vi "Liste-maker.vi"(1 "Path":path) -> (0 "Save Path":path)   [LabVIEW 2019]
panel:
  in  "load":bool
  in  "cancel":bool
  in  "Apperçu_ghost":string[][](table)=[["1", "NGC1", "1:00:00", "0:00:00", "2000"], ["2", "NGC2", "2:00:00", "-1:00:00", "2000"], ["3", "NGC3", "3:00:00", "-2:00:00", "2000"], ["4", "NGC4", "4:00:00", "-3:00:00", "2000"], ["5", "NGC5", "5:00:00", "-4:00:00", "2000"]]
  in  "i":string
  in  "reorder":bool
  in  "erase":bool
  in  "add":bool
  in  "Epoch":string
  in  "DEC":string
  in  "RA":string
  in  "Pseudonyme":string
  out "tmp_str":string
  in  "save":bool
  in  "stop":bool
  out "Apperçu":string[][](table)=[["1", "NGC1", "1:00:00", "0:00:00", "2000"], ["2", "NGC2", "2:00:00", "-1:00:00", "2000"], ["3", "NGC3", "3:00:00", "-2:00:00", "2000"], ["4", "NGC4", "4:00:00", "-3:00:00", "2000"], ["5", "NGC5", "5:00:00", "-4:00:00", "2000"]]
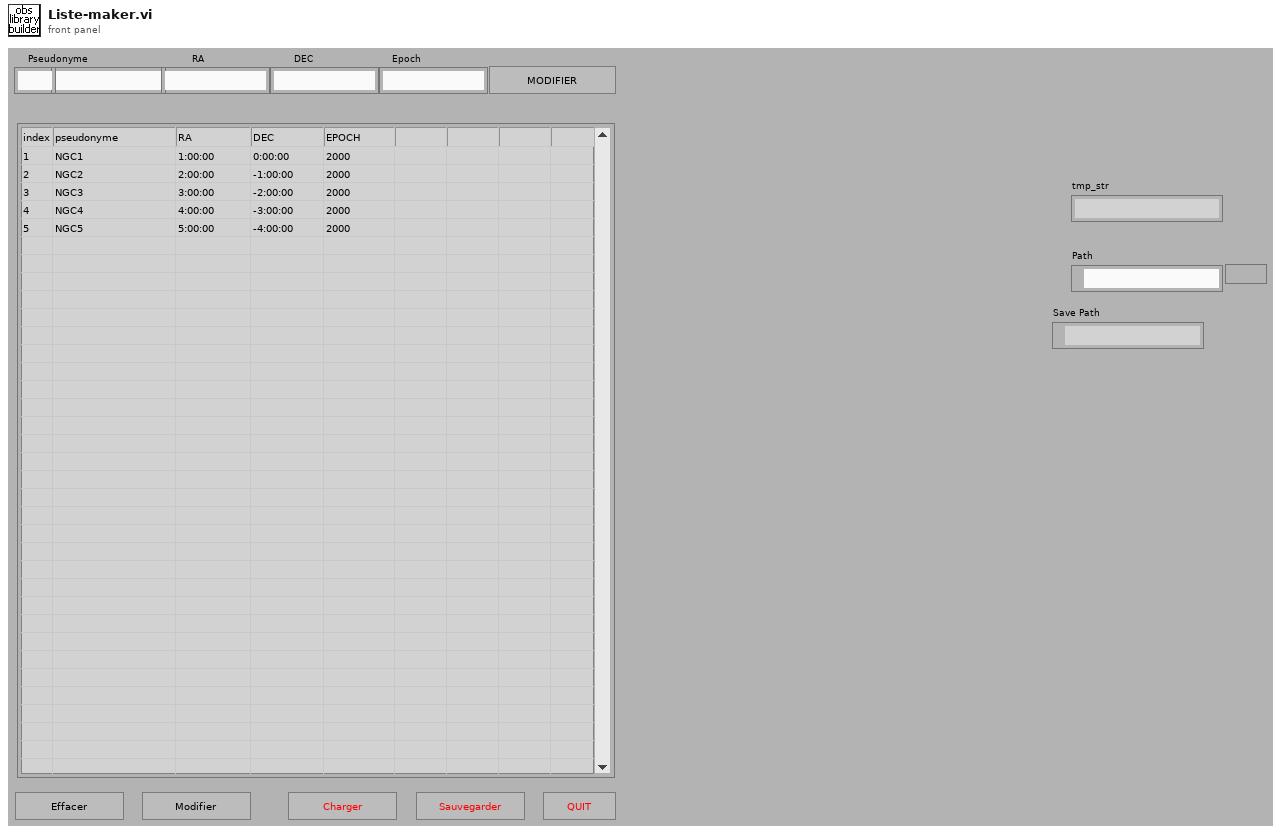
[diagram p1: front panel]
types:
  T1 = typedef "LVRowAndColumnTypeDef.ctl" = cluster{"Row":i32, "Column":i32}
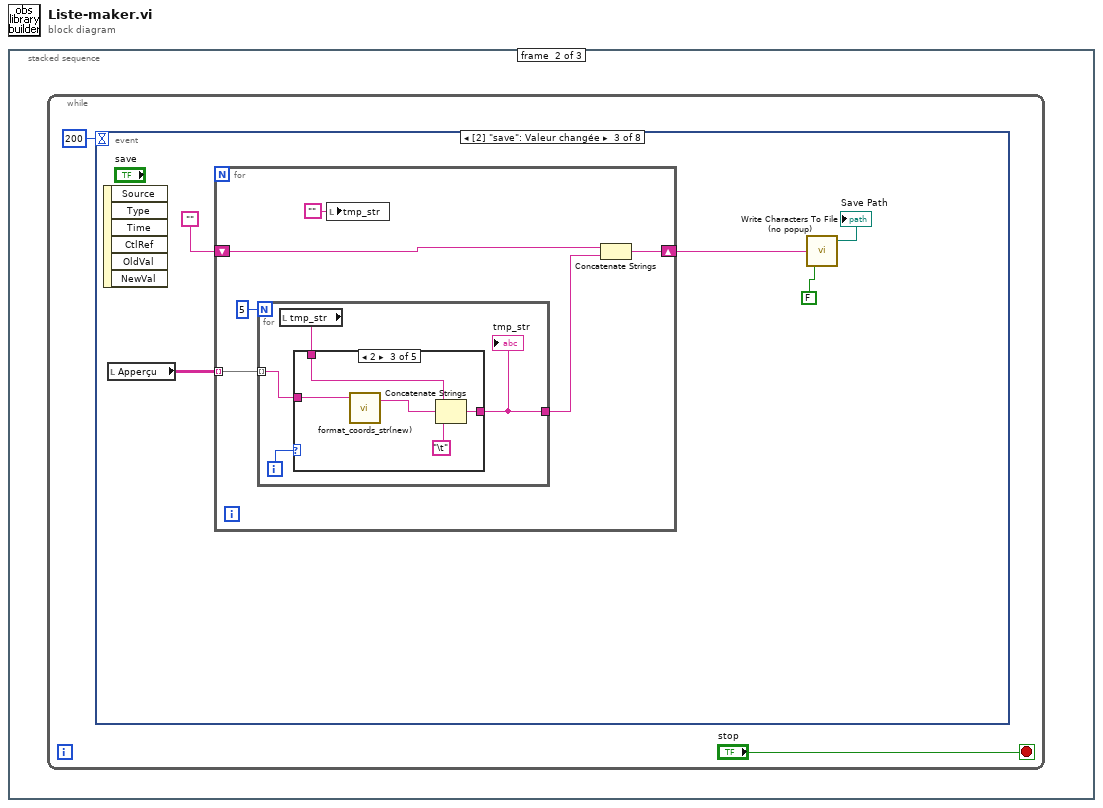
[diagram p0: block diagram]
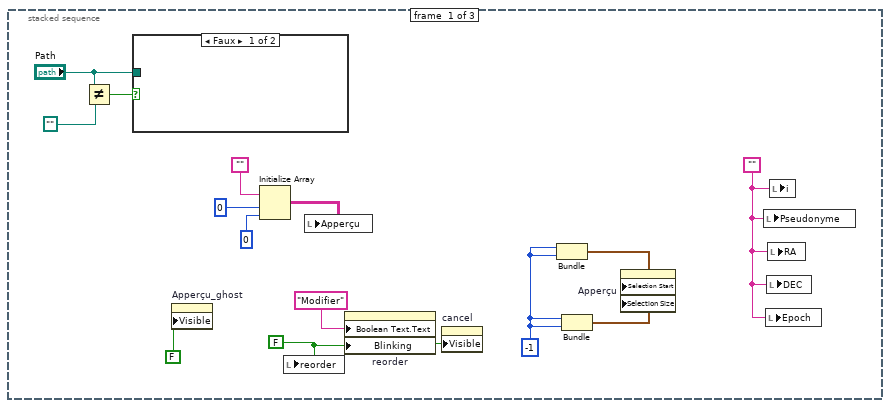
[diagram p2: hidden frame]
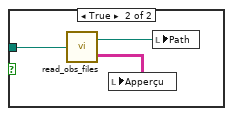
[diagram p3: hidden frame]
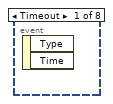
[diagram p4: hidden frame]
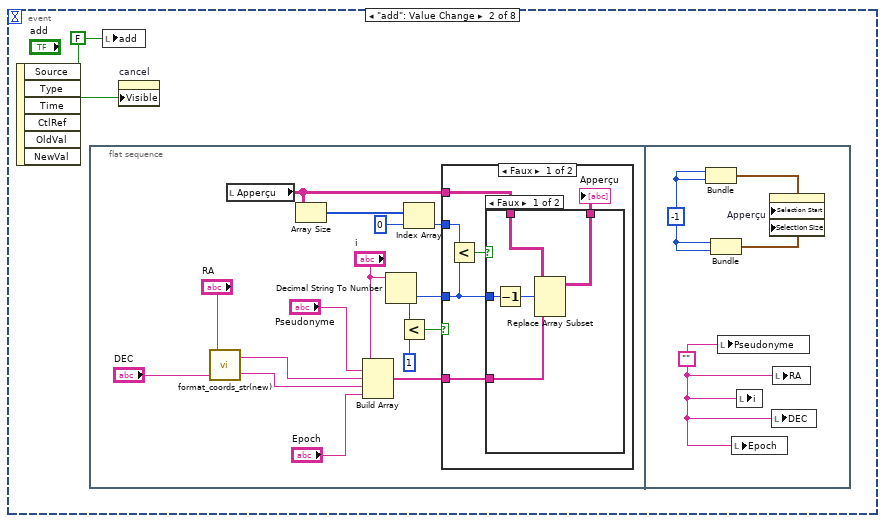
[diagram p5: hidden frame]
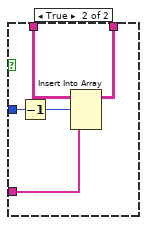
[diagram p6: hidden frame]
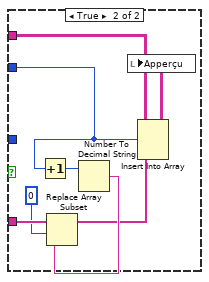
[diagram p7: hidden frame]
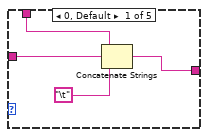
[diagram p8: hidden frame]
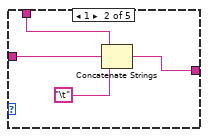
[diagram p9: hidden frame]
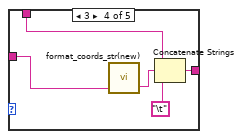
[diagram p10: hidden frame]
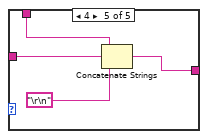
[diagram p11: hidden frame]
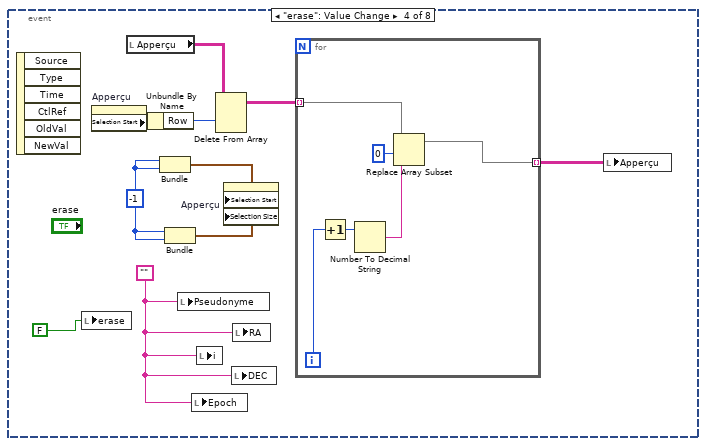
[diagram p12: hidden frame]
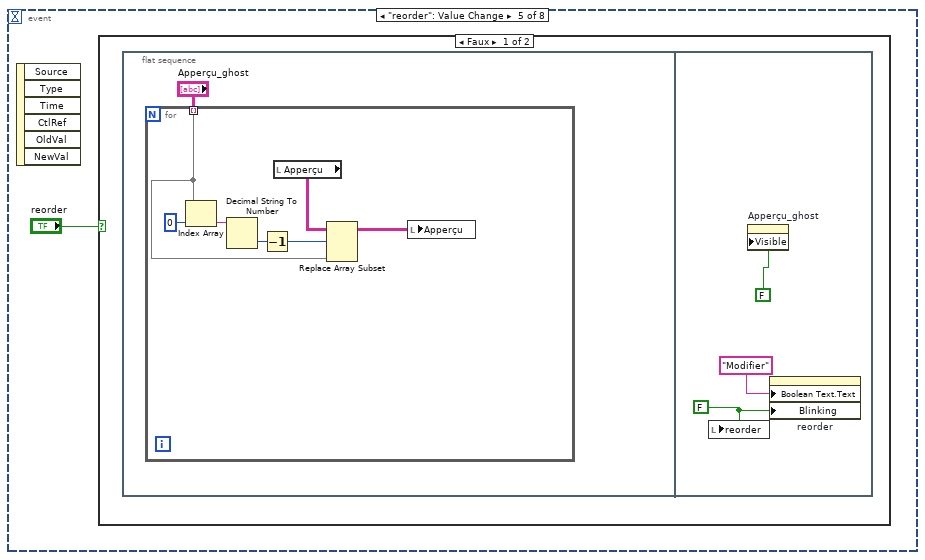
[diagram p13: hidden frame]
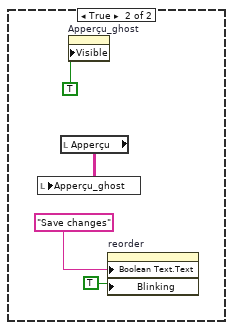
[diagram p14: hidden frame]
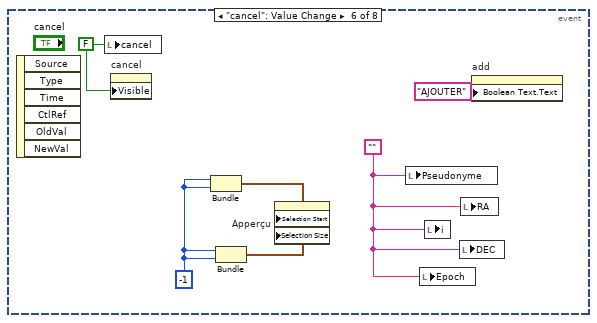
[diagram p15: hidden frame]
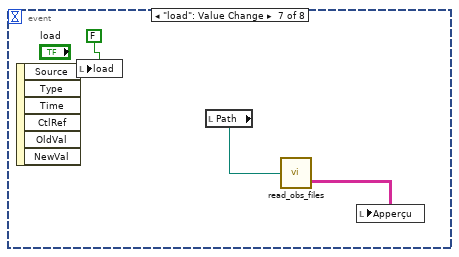
[diagram p16: hidden frame]
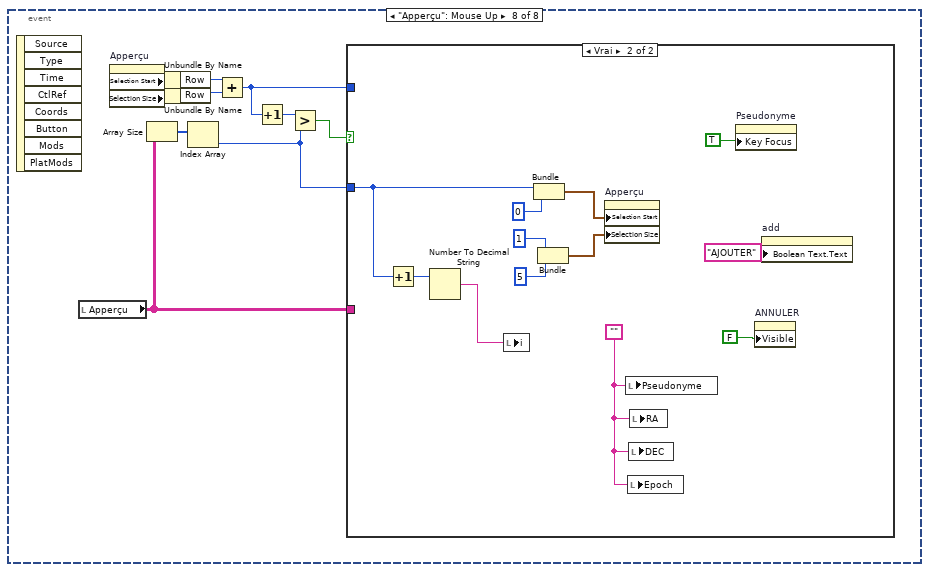
[diagram p17: hidden frame]
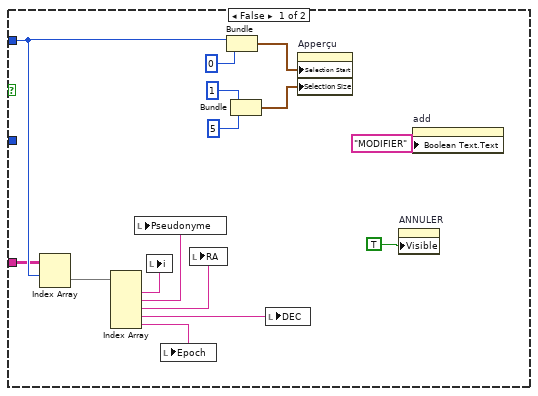
[diagram p18: hidden frame]
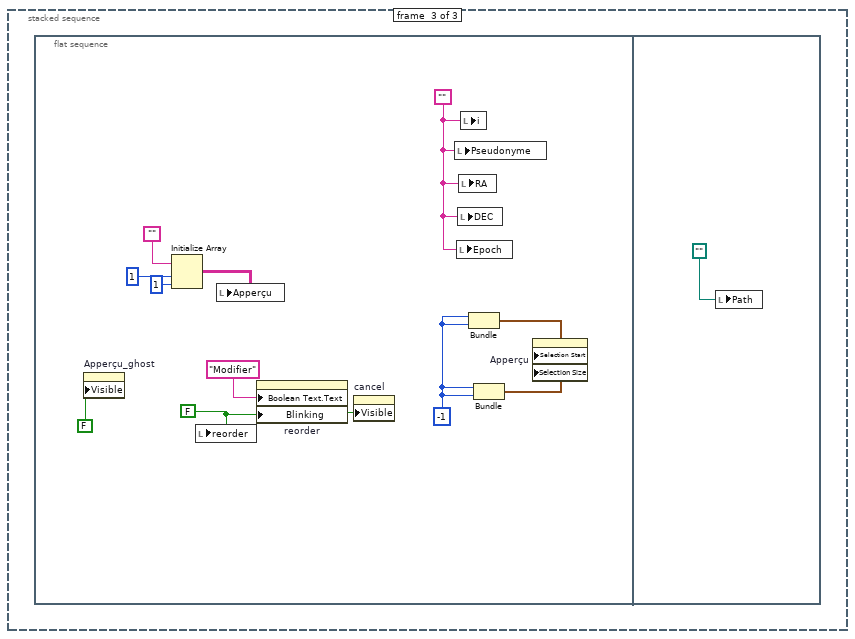
[diagram p19: hidden frame]
diagram:
  n1 = stacked-sequence {
    frame #0 {
      w4 = ""
      w8 = -1
      w7 = FALSE ("Visible")
      n2 = Not Equal?(x="Path", y=path "") -> (x != y?=w2:bool)
      n3 = case shown="Faux" w2 {
        tunnel: "Path" -> [_ w16]
        frame False {
        }
        frame True {
          n4 = call "read_obs_files.vi"("Path"=w16) -> ("path used"=w15:path, "Output Table"=w17:string[][])
          n5 = local write "Apperçu"(w17) -> ()
          n6 = local write "Path"(w15) -> ()
        }
      }
      n7 = property on="Apperçu_ghost" class="Tbl (strict)"("Visible"=FALSE) -> ()  [unwired: 2 in, 2 out]
      n8 = Initialize Array("", 0 ("dimension size"), 0 ("dimension size")) -> (w11:string[][])
      n9 = local write "reorder"(w7) -> ()
      n10 = local write "Apperçu"(w11) -> ()
      n11 = property on="reorder" class="Bool (strict)"("Boolean Text.Text"="Modifier" ("Caption.Text"), "Blinking"=w7) -> ()  [unwired: 2 in, 2 out]
      n12 = property on="cancel" class="Bool (strict)"("Visible"=w7) -> ()  [unwired: 2 in, 2 out]
      n13 = Bundle(w8, w8) -> (w10:cluster{i32, i32})  [unwired: 1 in]
      n14 = Bundle(w8, w8) -> (w9:cluster{i32, i32})  [unwired: 1 in]
      n15 = property on="Apperçu" class="Tbl (strict)"("Selection Start"=w10, "Selection Size"=w9) -> ()  [unwired: 2 in, 2 out]
      n16 = local write "Pseudonyme"(w4) -> ()
      n17 = local write "Epoch"(w4) -> ()
      n18 = local write "DEC"(w4) -> ()
      n19 = local write "RA"(w4) -> ()
      n20 = local write "i"(w4) -> ()
    }
    frame #1 {
      n21 = while {
        stop <- "stop" stop-if-true
        n22 = event shown="[2] \"save\": Valeur changée" {
          selector: _ -> [_ _ _ _ _ _ _ _]
          dyn-events: _ -> [_ _ _ _ _ _ _ _]
          timeout: 200 -> [_ _ _ _ _ _ _ _]
          event Timeout {
            n23 = event-data() -> ()  [unwired: 1 in, 2 out]
          }
          event "add": Value Change {
            w20 = FALSE
            n24 = event-data() -> ()  [unwired: 1 in, 6 out]
            n25 = flat-sequence {
              frame #0 {
                n26 = call "format_coords_str(new).vi"("DEC str"="DEC", "RA str"="RA") -> ("%s DEC"=w25:string, "%s RA"=w26:string)  [unwired: 1 in]
                n27 = local read "Apperçu"() -> (w24:string[][])
                n28 = Array Size(array=w24) -> (size(s)=w22:i32[])
                n29 = Build Array("i", "Pseudonyme", w26, w25, "Epoch") -> (w32:string[])
                n30 = Decimal String To Number(string="i") -> (number=w33:i32)  [unwired: 2 in, 1 out]
                n31 = Less?(x=w33, y=1) -> (x < y?=w35:bool)
                n32 = Index Array(array=w22, index=0) -> (element=w21:i32)
                n33 = case shown="Faux" w35 {
                  tunnel: w32 -> [w40 w57]
                  tunnel: w24 -> [w41 w58]
                  tunnel: w33 -> [w39 _]
                  tunnel: w21 -> [w37 w52]
                  frame False {
                    n34 = Less?(x=w37, y=w39) -> (x < y?=w38:bool)
                    n35 = case shown="Faux" w38 {
                      tunnel: w41 -> [w46 w50]
                      tunnel: w39 -> [w45 w48]
                      tunnel: w40 -> [w43 w51]
                      tunnel: [w42 w47] -> w36
                      frame False {
                        n36 = Decrement(x=w45) -> (x-1=w44:i32)
                        n37 = Replace Array Subset(array=w46, new element=w43, index (row)=w44) -> (w42:string[][])  [unwired: 1 in]
                      }
                      frame True {
                        n38 = Decrement(x=w48) -> (x-1=w49:i32)
                        n39 = Insert Into Array(array=w50, index (row)=w49, new element=w51) -> (w47:string[][])  [unwired: 1 in]
                      }
                    }
                    "Apperçu" <- w36
                  }
                  frame True {
                    n40 = Increment(x=w52) -> (x+1=w53:i32)
                    n41 = Number To Decimal String(number=w53) -> (decimal integer string=w56:string)  [unwired: 1 in]
                    n42 = Replace Array Subset(array=w57, new element=w56, index=0) -> (w55:string[])
                    n43 = Insert Into Array(array=w58, index (row)=w52, new element=w55) -> (w59:string[][])  [unwired: 1 in]
                    n44 = local write "Apperçu"(w59) -> ()
                  }
                }
              }
              frame #1 {
                w60 = ""
                w61 = -1
                n45 = Bundle(w61, w61) -> (w63:cluster{i32, i32})  [unwired: 1 in]
                n46 = Bundle(w61, w61) -> (w62:cluster{i32, i32})  [unwired: 1 in]
                n47 = local write "Pseudonyme"(w60) -> ()
                n48 = local write "Epoch"(w60) -> ()
                n49 = local write "i"(w60) -> ()
                n50 = property on="Apperçu" class="Tbl (strict)"("Selection Start"=w63, "Selection Size"=w62) -> ()  [unwired: 2 in, 2 out]
                n51 = local write "DEC"(w60) -> ()
                n52 = local write "RA"(w60) -> ()
              }
            }
            n53 = local write "add"(w20) -> ()
            n54 = property on="cancel" class="Bool (strict)"("Visible"=w20) -> ()  [unwired: 2 in, 2 out]
          }
          event "save": Value Change {
            n55 = event-data() -> ()  [unwired: 1 in, 6 out]
            n56 = local read "Apperçu"() -> (w68:string[][])
            n57 = for {
              tunnel: w68 -> [w74] mode=indexing
              shift-right: [w72] -> w66
              shift-left: "" -> [w70]
              n58 = for {
                N: 5 -> [_]
                tunnel: w74 -> [w76] mode=indexing
                tunnel: [w75] -> w73
                i -> [w78]
                n59 = local read "tmp_str"() -> (w77:string)
                n60 = case shown="2" w78 {
                  tunnel: w77 -> [w82 w86 w90 w95 w100]
                  tunnel: w76 -> [w81 w85 w89 w94 w99]
                  tunnel: [w79 w83 w91 w96 w98] -> w75
                  frame 0, Default {
                    n61 = Concatenate Strings(w82, w81, "\t") -> (w79:string)
                  }
                  frame 1 {
                    n62 = Concatenate Strings(w86, w85, "\t") -> (w83:string)
                  }
                  frame 2 {
                    n63 = call "format_coords_str(new).vi"("RA str"=w89) -> ("%s RA"=w87:string)  [unwired: 2 in, 1 out]
                    n64 = Concatenate Strings(w90, w87, "\t") -> (w91:string)
                  }
                  frame 3 {
                    n65 = call "format_coords_str(new).vi"("DEC str"=w94) -> ("%s DEC"=w93:string)  [unwired: 2 in, 1 out]
                    n66 = Concatenate Strings(w95, w93, "\t") -> (w96:string)
                  }
                  frame 4 {
                    n67 = Concatenate Strings(w100, w99, "\r\n") -> (w98:string)
                  }
                }
                "tmp_str" <- w75
              }
              n68 = local write "tmp_str"("") -> ()
              n69 = Concatenate Strings(w70, w73) -> (w72:string)
            }
            n70 = call "Write Characters To File (no popup).vi"("append to file? (new file:F)"=FALSE, "character string"=w66) -> ("new file path (Not A Path if cancelled)"=→"Save Path":path)  [unwired: 3 in]
          }
          event "erase": Value Change {
            w101 = -1
            w104 = ""
            n71 = event-data() -> ()  [unwired: 1 in, 6 out]
            n72 = local write "erase"(FALSE ("erase")) -> ()
            n73 = property on="Apperçu" class="Tbl (strict)"() -> ("Selection Start"=w109:T1)  [unwired: 2 in, 2 out]
            n74 = local read "Apperçu"() -> (w110:string[][])
            n75 = Unbundle By Name(w109) -> ("Row"=w108:i32)
            n76 = Bundle(w101, w101) -> (w103:cluster{i32, i32})  [unwired: 1 in]
            n77 = Bundle(w101, w101) -> (w102:cluster{i32, i32})  [unwired: 1 in]
            n78 = local write "Pseudonyme"(w104) -> ()
            n79 = local write "Epoch"(w104) -> ()
            n80 = local write "i"(w104) -> ()
            n81 = Delete From Array(array=w110, index (row)=w108) -> (array with subset deleted=w107:string[][])  [unwired: 2 in, 1 out]
            n82 = property on="Apperçu" class="Tbl (strict)"("Selection Start"=w103, "Selection Size"=w102) -> ()  [unwired: 2 in, 2 out]
            n83 = local write "DEC"(w104) -> ()
            n84 = local write "RA"(w104) -> ()
            n85 = for {
              tunnel: w107 -> [w115] mode=indexing
              tunnel: [w111] -> w106 mode=indexing
              i -> [w116]
              n86 = Increment(x=w116) -> (x+1=w113:i32)
              n87 = Number To Decimal String(number=w113) -> (decimal integer string=w112:string)  [unwired: 1 in]
              n88 = Replace Array Subset(array=w115, new element=w112, index=0) -> (w111:string[])
            }
            n89 = local write "Apperçu"(w106) -> ()
          }
          event "reorder": Value Change {
            n90 = event-data() -> ()  [unwired: 1 in, 6 out]
            n91 = case shown="Faux" "reorder" {
              frame False {
                n92 = flat-sequence {
                  frame #0 {
                    n93 = for {
                      tunnel: "Apperçu_ghost" -> [w119] mode=indexing
                      n94 = Index Array(array=w119, index=0) -> (element=w124:string)
                      n95 = Decimal String To Number(string=w124) -> (number=w122:i32)  [unwired: 2 in, 1 out]
                      n96 = Decrement(x=w122) -> (x-1=w121:i32)
                      n97 = local read "Apperçu"() -> (w123:string[][])
                      n98 = Replace Array Subset(array=w123, new element=w119, index (row)=w121) -> (w120:string[][])  [unwired: 1 in]
                      n99 = local write "Apperçu"(w120) -> ()
                    }
                  }
                  frame #1 {
                    w127 = FALSE ("Visible")
                    n100 = local write "reorder"(w127) -> ()
                    n101 = property on="Apperçu_ghost" class="Tbl (strict)"("Visible"=FALSE) -> ()  [unwired: 2 in, 2 out]
                    n102 = property on="reorder" class="Bool (strict)"("Boolean Text.Text"="Modifier" ("Caption.Text"), "Blinking"=w127) -> ()  [unwired: 2 in, 2 out]
                  }
                }
              }
              frame True {
                n103 = local read "Apperçu"() -> (w131:string[][])
                n104 = local write "Apperçu_ghost"(w131) -> ()
                n105 = property on="Apperçu_ghost" class="Tbl (strict)"("Visible"=TRUE) -> ()  [unwired: 2 in, 2 out]
                n106 = property on="reorder" class="Bool (strict)"("Boolean Text.Text"="Save changes" ("Caption.Text"), "Blinking"=TRUE) -> ()  [unwired: 2 in, 2 out]
              }
            }
          }
          event "cancel": Value Change {
            w133 = -1
            w138 = ""
            w136 = FALSE ("cancel")
            n107 = event-data() -> ()  [unwired: 1 in, 6 out]
            n108 = local write "cancel"(w136) -> ()
            n109 = property on="cancel" class="Bool (strict)"("Visible"=w136) -> ()  [unwired: 2 in, 2 out]
            n110 = Bundle(w133, w133) -> (w135:cluster{i32, i32})  [unwired: 1 in]
            n111 = Bundle(w133, w133) -> (w134:cluster{i32, i32})  [unwired: 1 in]
            n112 = property on="Apperçu" class="Tbl (strict)"("Selection Start"=w135, "Selection Size"=w134) -> ()  [unwired: 2 in, 2 out]
            n113 = local write "Pseudonyme"(w138) -> ()
            n114 = local write "Epoch"(w138) -> ()
            n115 = local write "i"(w138) -> ()
            n116 = local write "DEC"(w138) -> ()
            n117 = local write "RA"(w138) -> ()
            n118 = property on="add" class="Bool (strict)"("Boolean Text.Text"="AJOUTER") -> ()  [unwired: 2 in, 2 out]
          }
          event "load": Value Change {
            n119 = event-data() -> ()  [unwired: 1 in, 6 out]
            n120 = local write "load"(FALSE ("load")) -> ()
            n121 = local read "Path"() -> (w139:path)
            n122 = call "read_obs_files.vi"("Path"=w139) -> ("Output Table"=w140:string[][])  [unwired: 1 out]
            n123 = local write "Apperçu"(w140) -> ()
          }
          event "Apperçu": Mouse Up {
            n124 = event-data() -> ()  [unwired: 1 in, 8 out]
            n125 = local read "Apperçu"() -> (w146:string[][])
            n126 = property on="Apperçu" class="Tbl (strict)"() -> ("Selection Start"=w151:T1, "Selection Size"=w150:T1)  [unwired: 2 in, 2 out]
            n127 = Array Size(array=w146) -> (size(s)=w147:i32[])
            n128 = Unbundle By Name(w151) -> ("Row"=w148:i32)
            n129 = Unbundle By Name(w150) -> ("Row"=w149:i32)
            n130 = Index Array(array=w147) -> (element=w142:i32)  [unwired: 1 in]
            n131 = Add(x=w148, y=w149) -> (x+y=w144:i32)
            n132 = Increment(x=w144) -> (x+1=w145:i32)
            n133 = Greater?(x=w145, y=w142) -> (0:w143:bool)
            n134 = case shown="Vrai" w143 {
              tunnel: w144 -> [w161 _]
              tunnel: w146 -> [w152 _]
              tunnel: w142 -> [_ w173]
              frame False {
                n135 = Index Array(array=w152, index (row)=w161) -> (element=w160:string[])  [unwired: 1 in]
                n136 = Index Array(array=w160) -> (element #1=w155:string, element #2=w159:string, element #3=w158:string, element #4=w157:string, element #5=w156:string)  [unwired: 5 in]
                n137 = local write "Pseudonyme"(w159) -> ()
                n138 = local write "i"(w155) -> ()
                n139 = local write "Epoch"(w156) -> ()
                n140 = local write "RA"(w158) -> ()
                n141 = Bundle(w161, 0) -> (w163:cluster{i32, i32})  [unwired: 1 in]
                n142 = Bundle(1, 5) -> (w162:cluster{i32, i32})  [unwired: 1 in]
                n143 = local write "DEC"(w157) -> ()
                n144 = property on="Apperçu" class="Tbl (strict)"("Selection Start"=w163, "Selection Size"=w162) -> ()  [unwired: 2 in, 2 out]
                n145 = property on="ANNULER" class="Bool (strict)"("Visible"=TRUE) -> ()  [unwired: 2 in, 2 out]
                n146 = property on="add" class="Bool (strict)"("Boolean Text.Text"="MODIFIER") -> ()  [unwired: 2 in, 2 out]
              }
              frame True {
                w172 = ""
                n147 = Increment(x=w173) -> (x+1=w171:i32)
                n148 = Number To Decimal String(number=w171) -> (decimal integer string=w169:string)  [unwired: 1 in]
                n149 = local write "i"(w169) -> ()
                n150 = Bundle(w173, 0) -> (w175:cluster{i32, i32})  [unwired: 1 in]
                n151 = Bundle(1, 5) -> (w174:cluster{i32, i32})  [unwired: 1 in]
                n152 = property on="Apperçu" class="Tbl (strict)"("Selection Start"=w175, "Selection Size"=w174) -> ()  [unwired: 2 in, 2 out]
                n153 = local write "Pseudonyme"(w172) -> ()
                n154 = local write "Epoch"(w172) -> ()
                n155 = local write "DEC"(w172) -> ()
                n156 = local write "RA"(w172) -> ()
                n157 = property on="Pseudonyme" class="Ch"("Key Focus"=TRUE) -> ()  [unwired: 2 in, 2 out]
                n158 = property on="ANNULER" class="Bool (strict)"("Visible"=FALSE) -> ()  [unwired: 2 in, 2 out]
                n159 = property on="add" class="Bool (strict)"("Boolean Text.Text"="AJOUTER") -> ()  [unwired: 2 in, 2 out]
              }
            }
          }
        }
      }
    }
    frame #2 {
      n160 = flat-sequence {
        frame #0 {
          w179 = ""
          w183 = -1
          w182 = FALSE ("Visible")
          n161 = property on="Apperçu_ghost" class="Tbl (strict)"("Visible"=FALSE) -> ()  [unwired: 2 in, 2 out]
          n162 = Initialize Array("", 1 ("dimension size"), 1 ("dimension size")) -> (w186:string[][])
          n163 = local write "reorder"(w182) -> ()
          n164 = local write "Apperçu"(w186) -> ()
          n165 = property on="reorder" class="Bool (strict)"("Boolean Text.Text"="Modifier" ("Caption.Text"), "Blinking"=w182) -> ()  [unwired: 2 in, 2 out]
          n166 = property on="cancel" class="Bool (strict)"("Visible"=w182) -> ()  [unwired: 2 in, 2 out]
          n167 = local write "Pseudonyme"(w179) -> ()
          n168 = local write "Epoch"(w179) -> ()
          n169 = local write "DEC"(w179) -> ()
          n170 = local write "RA"(w179) -> ()
          n171 = local write "i"(w179) -> ()
          n172 = Bundle(w183, w183) -> (w185:cluster{i32, i32})  [unwired: 1 in]
          n173 = Bundle(w183, w183) -> (w184:cluster{i32, i32})  [unwired: 1 in]
          n174 = property on="Apperçu" class="Tbl (strict)"("Selection Start"=w185, "Selection Size"=w184) -> ()  [unwired: 2 in, 2 out]
        }
        frame #1 {
          n175 = local write "Path"(path "") -> ()
        }
      }
    }
  }
